vi "updateFromLandmarks.vi"(8 "landmarkNumber":i32, 9 "measurement":dbl[](array[numeric]), 10 "P":dbl[][](array[numeric]), 11 "X":dbl[](array[numeric])) -> (2 "P out":dbl[][](array[numeric]), 3 "X out":dbl[](array[numeric]))   [LabVIEW 2009, in "LV_SLAM.lvlib"]
uses:
  LV_SLAM.lvlib
  <vilib>/Analysis/Matrix/Datatypes/RealMatrix.ctl
  <vilib>/Analysis/Matrix/Numeric/Multiply/Multiply - RM,RM.vi
  <vilib>/Analysis/Matrix/Numeric/Subtract/Subtract - RM,RM.vi
  <vilib>/Analysis/baseanly.llb/Real Inverse Matrix.vi
  <vilib>/Analysis/Matrix/Numeric/Add/Add - RM,RM.vi
  <vilib>/Analysis/Matrix/Numeric/Conversions/Array To Matrix.vi
  <vilib>/Analysis/Matrix/Numeric/Conversions/Array To Matrix - RA2.vi
  <vilib>/Analysis/Matrix/NI_Matrix.lvlib
  <vilib>/Analysis/NI_AALBase.lvlib
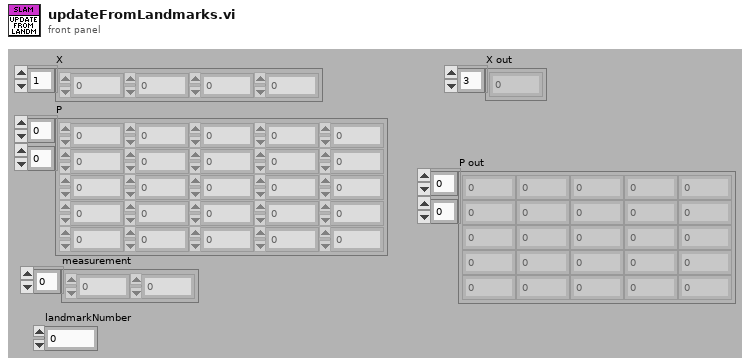
[diagram p1: front panel]
types:
  T1 = typedef "NI_Matrix.lvlib/RealMatrix.ctl" = dbl[][]
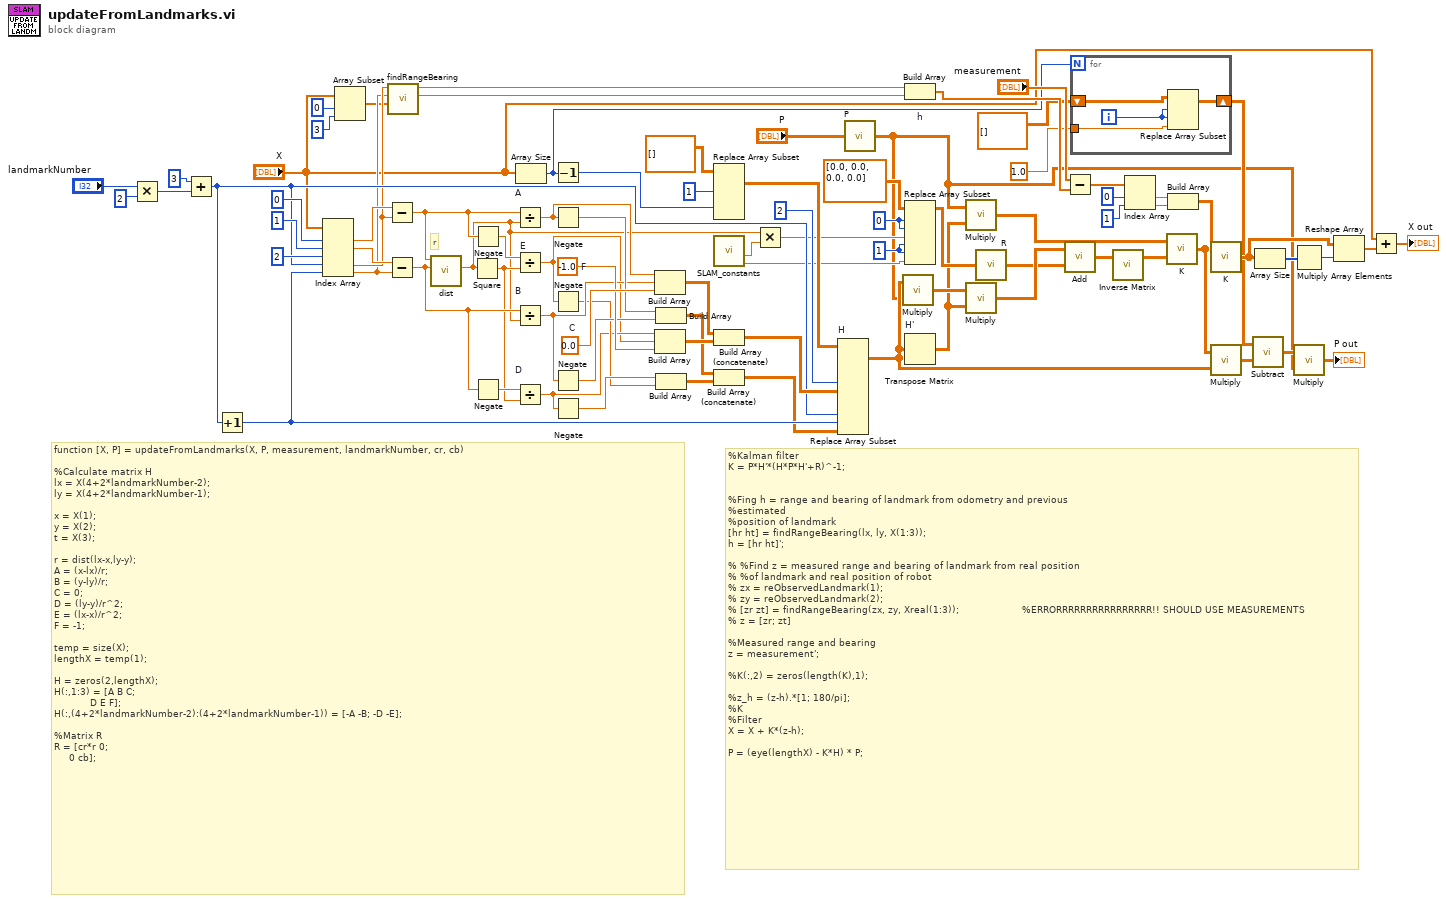
[diagram p0: block diagram]
diagram:
  w46 = 1 ("index (row)")
  w47 = 0 ("index (row)")
  w67 = -1.0  # F
  w68 = 0.0  # C
  # "%Kalman filter\nK = P*H'*(H*P*H'+R)^-1;\n\n\n%Fing h = range and bearing of landmark from odometry and previous\n%estimated\n%position of landmark\n[hr ht] = findRangeBearing(lx, ly, X(1:3));\nh = [hr ht]';\n\n% %Find z = measured range and bearing of landmark from real position\n% %of landmark and real position of robot\n% zx = reObservedLandmark(1);\n% zy = reObservedLandmark(2);\n% [zr zt] = findRangeBearing(zx, zy, Xreal(1:3));                     %ERRORRRRRRRRRRRRRRRR!! SHOULD USE MEASUREMENTS\n% z = [zr; zt]\n\n%Measured range and bearing\nz = measurement';\n\n%K(:,2) = zeros(length(K),1);\n\n%z_h = (z-h).*[1; 180/pi];\n%K\n%Filter\nX = X + K*(z-h);\n\nP = (eye(lengthX) - K*H) * P;"
  # "r"
  # "function [X, P] = updateFromLandmarks(X, P, measurement, landmarkNumber, cr, cb)\n\n%Calculate matrix H\nlx = X(4+2*landmarkNumber-2);\nly = X(4+2*landmarkNumber-1);\n\nx = X(1);\ny = X(2);\nt = X(3);\n\nr = dist(lx-x,ly-y);\nA = (x-lx)/r;\nB = (y-ly)/r;\nC = 0;\nD = (ly-y)/r^2;\nE = (lx-x)/r^2;\nF = -1;\n\ntemp = size(X);\nlengthX = temp(1);\n\nH = zeros(2,lengthX);\nH(:,1:3) = [A B C;\n            D E F];\nH(:,(4+2*landmarkNumber-2):(4+2*landmarkNumber-1)) = [-A -B; -D -E];\n\n%Matrix R\nR = [cr*r 0;\n     0 cb];"
  n1 = Multiply(x="landmarkNumber", y=2) -> (x*y=w84:i32)
  n2 = Add(x=3 ("landmarkNumber"), y=w84) -> (x+y=w61:i32)
  n3 = Increment(x=w61) -> (x+1=w60:i32)
  n4 = Index Array(array="X", index #1=0 ("index"), index #2=1 ("index"), index #3=2 ("index"), index #4=w61, index #5=w60) -> (element #1=w77:dbl, element #2=w76:dbl, element #4=w32:dbl, element #5=w31:dbl)  [unwired: 1 out]
  n5 = Array Subset(array="X", index=0, length=3) -> (w28:dbl[])
  n6 = Subtract(x=w77, y=w32) -> (x-y=w73:dbl)
  n7 = Subtract(x=w76, y=w31) -> (x-y=w75:dbl)
  n8 = call "findRangeBearing.vi"("X"=w28, "ly"=w31, "lx"=w32) -> ("tt"=w26:dbl, "rr"=w27:dbl)  [unwired: 7 in]
  n9 = call "dist.vi"("y"=w75, "x"=w73) -> ("d"=w41:dbl)  [unwired: 9 in]
  n10 = Square(x=w41) -> (x^2=w71:dbl)
  n11 = Negate(x=w73) -> (-x=w72:dbl)
  n12 = Negate(x=w75) -> (-x=w74:dbl)
  n13 = Divide "A"(x=w73, y=w41) -> (x/y=w55:dbl)
  n14 = Divide "E"(x=w72, y=w71) -> (x/y=w49:dbl)
  n15 = Divide "B"(x=w75, y=w41) -> (x/y=w54:dbl)
  n16 = Divide "D"(x=w74, y=w71) -> (x/y=w50:dbl)
  n17 = Array Size(array="X") -> (size(s)=w8:i32)
  n18 = Decrement(x=w8) -> (x-1=w11:i32)
  n19 = Negate(x=w55) -> (-x=w56:dbl)
  n20 = Negate(x=w49) -> (-x=w51:dbl)
  n21 = Negate(x=w54) -> (-x=w53:dbl)
  n22 = Negate(x=w50) -> (-x=w52:dbl)
  n23 = Build Array(w55, w54, w68) -> (w66:T1)
  n24 = Build Array(w50, w49, w67) -> (w65:T1)
  n25 = Build Array(w56, w53) -> (w59:T1)
  n26 = Build Array(w52, w51) -> (w58:T1)
  n27 = Replace Array Subset(array=T1 [] ("matrix"), index (dim 1)=1 ("row N"), index (dim 3)=w11) -> (w64:T1)  [unwired: 3 in]
  n28 = call "SLAM_constants.vi"() -> ("cb"=w42:dbl, "cr"=w43:dbl)  [unwired: 7 in, 3 out]
  n29 = Build Array (concatenate)(w66, w65) -> (w63:T1)
  n30 = Build Array (concatenate)(w59, w58) -> (w57:T1)
  n31 = Multiply(x=w41, y=w43) -> (x*y=w45:dbl)
  n32 = Replace Array Subset "H"(array=w64, new element #1=w63, index (dim 3) #1=2 ("column N"), new element #2=w57, index (dim 2) #2=w61, index (dim 3) #2=w60) -> (w6:T1)  [unwired: 5 in]
  n33 = call-poly "P"("Real 2D Array"="P") -> ("Real Matrix"=w2:T1)
  n34 = call-poly <vilib>:"Multiply.vi"("Real Matrix B"=w2, "Real Matrix A"=w6) -> ("A * B"=w39:T1)
  n35 = Build Array "h"(w27, w26) -> (w24:dbl[])
  n36 = Replace Array Subset(array=dbl[][] [[0.0, 0.0], [0.0, 0.0]] ("P"), new element #1=w45, index (row) #1=w47, index (col) #1=w47, new element #2=w42, index (row) #2=w46, index (col) #2=w46) -> (w44:dbl[][])
  n37 = Transpose Matrix "H'"(1:w6) -> (0:w38:T1)
  n38 = call-poly <vilib>:"Multiply.vi"("Real Matrix B"=w38, "Real Matrix A"=w2) -> ("A * B"=w34:T1)
  n39 = call-poly <vilib>:"Multiply.vi"("Real Matrix B"=w38, "Real Matrix A"=w39) -> ("A * B"=w37:T1)
  n40 = call-poly "R"("Real 2D Array"=w44) -> ("Real Matrix"=w36:T1)
  n41 = Subtract(x="measurement", y=w24) -> (x-y=w23:dbl[])
  n42 = call-poly <vilib>:"Add.vi"("Real Matrix B"=w36, "Real Matrix A"=w37) -> ("A + B"=w35:T1)
  n43 = for {
    N: w8 -> [_]
    shift-right: [w87] -> w4
    shift-left: T1 [] ("matrix") -> [w88]
    tunnel: 1.0 ("new diagonal/fill element") -> [w86]
    i -> [w85]
    n44 = Replace Array Subset(array=w88, new element=w86, index (row)=w85, index (col)=w85) -> (w87:T1)
  }
  n45 = call-poly <vilib>:"Inverse Matrix.vi"("Input Matrix"=w35) -> ("Inverse Matrix"=w33:T1)  [unwired: 1 in, 1 out]
  n46 = Index Array(array=w23, index #1=0 ("index"), index #2=1 ("index")) -> (element #1=w20:dbl, element #2=w19:dbl)
  n47 = call-poly "K"("Real Matrix B"=w33, "Real Matrix A"=w34) -> ("A * B"=w7:T1)
  n48 = Build Array(w20, w19) -> (w18:T1)
  n49 = call-poly "K"("Real Matrix B"=w18, "Real Matrix A"=w7) -> ("A * B"=w17:T1)
  n50 = call-poly <vilib>:"Multiply.vi"("Real Matrix B"=w6, "Real Matrix A"=w7) -> ("A * B"=w5:T1)
  n51 = call-poly <vilib>:"Subtract.vi"("Real Matrix B"=w5, "Real Matrix A"=w4) -> ("A - B"=w3:T1)
  n52 = Array Size(array=w17) -> (size(s)=w16:i32[])
  n53 = Multiply Array Elements(1:w16) -> (0:w15:i32)
  n54 = call-poly <vilib>:"Multiply.vi"("Real Matrix B"=w2, "Real Matrix A"=w3) -> ("A * B"=→"P out":T1)
  n55 = Reshape Array(w17, w15) -> (w14:dbl[])
  n56 = Add(x="X", y=w14) -> (x+y=→"X out":dbl[])
